vi "VoltsToTemperature.vi"(0 "Voltage / V":dbl, 4 "Rset":dbl=10000.0, 5 "Vref":dbl=1.0, 6 "Rgain":dbl=100000.0 format="%#_13g") -> (1 "Temperature / C":dbl=25.0 format="%0.2f")   [LabVIEW 2014]
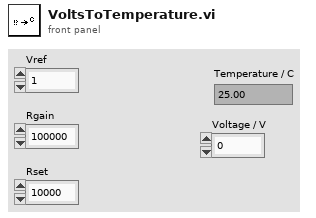
[diagram p1: front panel]
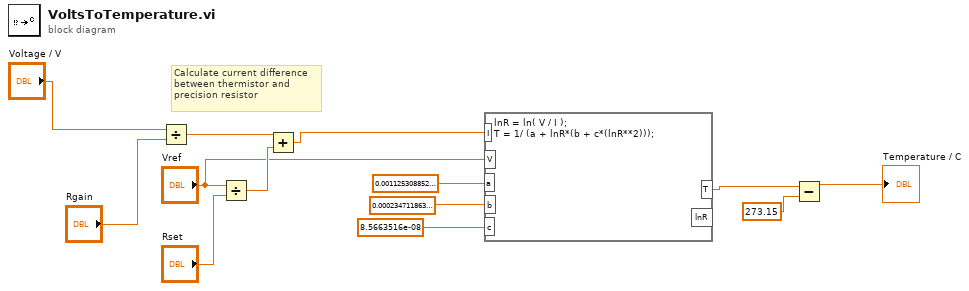
[diagram p0: block diagram]
diagram:
  # "Calculate current difference\nbetween thermistor and\nprecision resistor"
  n1 = Divide(x="Voltage / V", y="Rgain") -> (x/y=w12:dbl)
  n2 = Divide(x="Vref", y="Rset") -> (x/y=w10:dbl)
  n3 = Add(x=w12, y=w10) -> (x+y=w8:dbl)
  n4 = formula code="lnR = ln( V / I );\nT = 1/ (a + lnR*(b + c*(lnR**2)));"("V"="Vref", "a"=0.001125308852122, "b"=0.000234711863267, "c"=8.5663516e-08, "I"=w8) -> ("T"=w7:dbl)  [unwired: 1 out]
  n5 = Subtract(x=w7, y=273.15) -> (x-y=→"Temperature / C":dbl)
